vi "1.4odb.vi"() -> ()   [LabVIEW 2020]
uses:
  <vilib>/measure/maspectr.llb/FFT Power Spectrum and PSD for 1 Chan.vi
  <vilib>/measure/NI_MAPro.lvlib
panel:
  in  "Logarithmic Scale":bool
  in  "Window":u32(ring)=1 items=["Rectangle"=0, "Hanning"=1, "Hamming"=2, "Blackman-Harris"=3, "Exact Blackman"=4, "Blackman"=5, "Flat Top"=6, "4 Term B-Harris "=7, "7 Term B-Harris"=8, "Low Sidelobe"=9, "Blackman Nuttall"=11, "Triangle"=30, "Bartlett-Hanning"=31, "Bohman"=32, "Parzen"=33, "Welch"=34, "Kaiser"=60, "Dolph-Chebyshev"=61, "Gaussian"=62]
  out "Signal Waveform":waveform(dbl)(graph)
  out "Frequency Spectrum":cluster{"f0":dbl, "df":dbl, "magnitude":dbl[]}(graph)
  in  "stop":bool
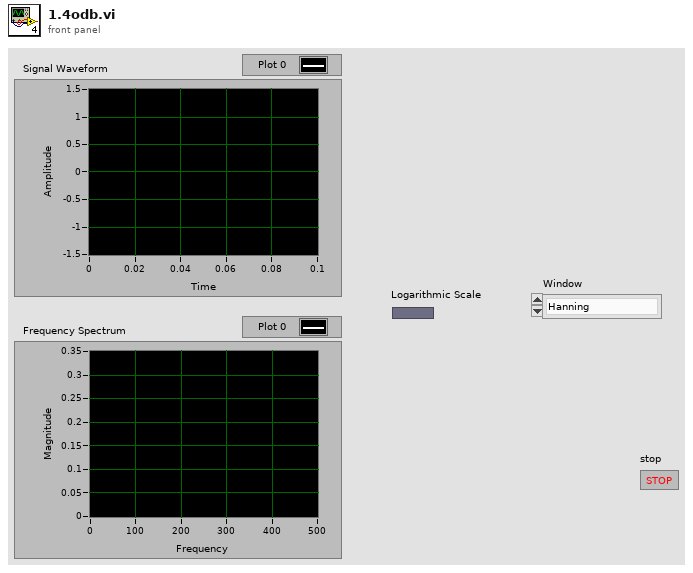
[diagram p1: front panel]
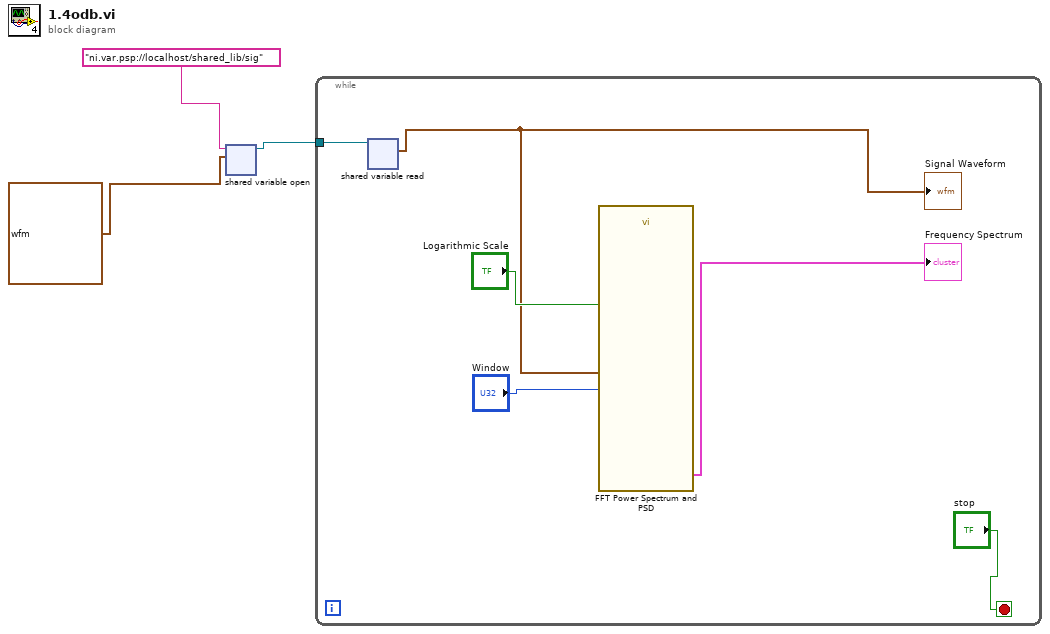
[diagram p0: block diagram]
diagram:
  n1 = shared-variable-open("ni.var.psp://localhost/shared_lib/sig", waveform(dbl) {"t0"=timestamp(0 s since 1904-01-01), "dt"=1.0, "Y"=[]} ("Waveform")) -> (w3:refnum<k21>)  [unwired: 2 in, 1 out]
  n2 = while {
    tunnel: w3 -> [w5]
    stop <- "stop" stop-if-true
    n3 = shared-variable-read(w5) -> (w4:waveform(dbl))  [unwired: 1 in, 3 out]
    "Signal Waveform" <- w4
    n4 = call-poly <vilib>:"FFT Power Spectrum and PSD.vi"("dB On (F)"="Logarithmic Scale", "window"="Window", "time signal"=w4) -> ("Power Spectrum / PSD"=→"Frequency Spectrum":cluster{"f0":dbl, "df":dbl, "magnitude":dbl[]})  [unwired: 5 in, 3 out]
  }
